vi "Read.vi"(11 "StringValue in":refnum<class "StringValue.lvclass">) -> (2 "Value":string)   [LabVIEW 2020, in "Volatus.lvlib" / "StringValue.lvclass"]
uses:
  StringValue.lvclass
  StringValue.lvclass/StringValue.ctl
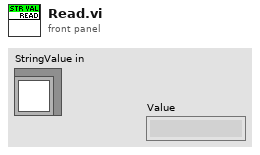
[diagram p1: front panel]
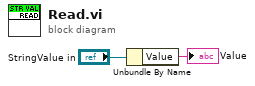
[diagram p0: block diagram]
diagram:
  n1 = Unbundle By Name("StringValue in") -> ("Value"=→"Value":string)
